vi "WriteMemory_u16.vi"(8 "Error In":errorcluster, 9 "Offset":T1, 10 "Data In":u16[][][](array[numeric]), 11 "Memory Object In":T2={"Device ID"=0, "Memeroy ID"=0, "Dimension"={"Depth"=1, "Height"=1, "Width"=1}, "Memory Type"=enum."32f"} {"Dimension"."Width" min=1; "Dimension"."Height" min=1; "Dimension"."Depth" min=1}) -> (0 "Error Out":errorcluster, 3 "Memory Object Out":T2={"Device ID"=0, "Memeroy ID"=0, "Dimension"={"Depth"=1, "Height"=1, "Width"=1}, "Memory Type"=enum."32f"} {"Dimension"."Width" min=1; "Dimension"."Height" min=1; "Dimension"."Depth" min=1})   [LabVIEW 2012, in "OpenCLV x64.lvlib"]
doc: "Writes 3D u16 memory from the host to the device."
uses:
  OpenCLV x64.lvlib
  Controls/Memory Object.ctl
  Controls/Device ID.ctl
  Controls/Memory ID.ctl
  User Controls/Array Dimensions.ctl
  Controls/Memory Type.ctl
  User Controls/Offset.ctl
  Error Checking/Add Error Functional Global.vi
panel:
  out "ms":dbl
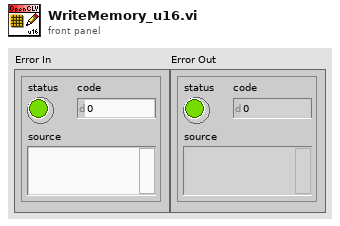
[diagram p1: front panel]
types:
  T1 = typedef "Offset.ctl" = cluster{"X":u64, "Y":u64, "Z":u64}
  T2 = typedef "OpenCLV x64.lvlib/Memory Object.ctl" = cluster{"Device ID":T3, "Memeroy ID":T4, "Dimension":T5, "Memory Type":T6}
  T3 = typedef "OpenCLV x64.lvlib/Device ID.ctl" = u64
  T4 = typedef "OpenCLV x64.lvlib/Memory ID.ctl" = u64
  T5 = typedef "Array Dimensions.ctl" = cluster{"Depth":u64, "Height":u64, "Width":u64}
  T6 = typedef "OpenCLV x64.lvlib/Memory Type.ctl" = enum16{"32f", "u8", "i8", "u16", "i16", "u32", "i32", "64f"}
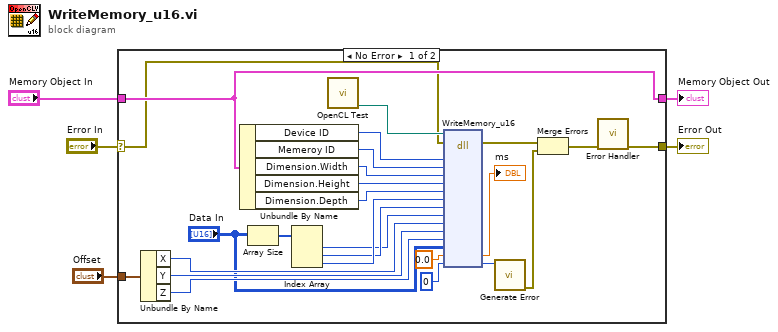
[diagram p0: block diagram]
diagram:
  n1 = case shown="No Error" "Error In" {
    selector: "Error In" -> [w6 w32]
    tunnel: [w12 w32] -> w4
    tunnel: "Memory Object In" -> [w15 w31]
    tunnel: "Offset" -> [w24 _]
    tunnel: [w15 w31] -> w1
    frame No Error {
      n2 = Unbundle By Name(w24) -> ("X"=w21:u64, "Y"=w22:u64, "Z"=w23:u64)
      n3 = Unbundle By Name(w15) -> ("Device ID"=w16:T3, "Memeroy ID"=w17:T4, "Dimension.Width"=w18:u64, "Dimension.Height"=w19:u64, "Dimension.Depth"=w20:u64)
      n4 = Array Size(array="Data In") -> (size(s)=w10:i32[])
      n5 = Index Array(array=w10) -> (element #1=w7:i32, element #2=w8:i32, element #3=w9:i32)  [unwired: 3 in]
      n6 = call "OpenCL Test.vi"() -> ("DLL To Use"=w29:path)  [unwired: 11 in]
      n7 = dll-call lib="D:/OpenCLV/trunk/OpenCLV_x64_1.0/OpenCLV_x64.dll" fn="WriteMemory_u16"(path in=w29, error in=w6, "Labview Device"=w16, "Device Memory"=w17, "DevWidth"=w18, "DevHeight"=w19, "DevDepth"=w20, "HostWidth"=w9, "HostHeight"=w8, "HostDepth"=w7, "X Offset"=w21, "Y Offset"=w22, "Z Offset"=w23, "Data"="Data In", "Time in ms"=0.0 ("Time"), "Error"=0) -> (error out=w14:errorcluster, "Time in ms"=→"ms":dbl, "Error"=w26:i32)  [unwired: 14 in, 1 out]
      n8 = call "Generate Error.vi"("Error"=w26) -> ("error out"=w30:errorcluster)  [unwired: 10 in]
      n9 = Merge Errors(w14, w30) -> (w13:errorcluster)
      n10 = call-poly "Error Handler.vi"("Error In"=w13) -> ("Error Out"=w12:errorcluster)  [unwired: 10 in]
    }
    frame Error {
    }
  }
  "Error Out" <- w4
  "Memory Object Out" <- w1
